vi "EndTest_WithTime_DurationIsSet.vi"() -> (0 "error out":errorcluster)   [LabVIEW 2017, in "ResultTreeListenerTest.lvlib"]
uses:
  ResultTreeListenerTest.lvlib
  ResultTreeListener/ResultTreeListener.lvclass
  ResultTree/ResultTree.lvclass
  Support/FakeTestCase/FakeTestCase.lvclass
  C:/Users/de200256/Code/neuperger/lvunit/Test/Test.lvclass
  275d98eb-69a7-4435-8809-2af3ffd1cf1d.vi
panel:
  in  "Tree":string(tree)
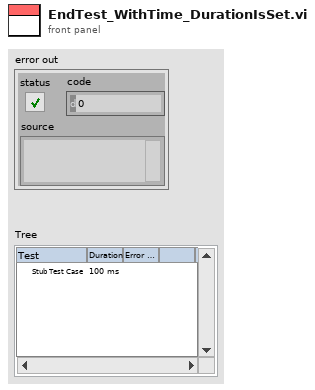
[diagram p1: front panel]
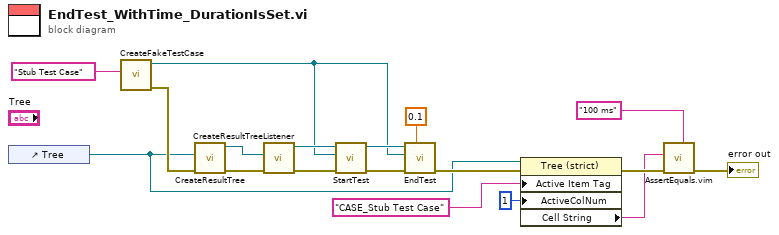
[diagram p0: block diagram]
diagram:
  n1 = control-ref of="Tree"() -> (w5:refnum<vi>)
  n2 = call "CreateFakeTestCase.vi"("Name"="Stub Test Case") -> ("error out"=w10:errorcluster, "FakeTestCase out"=w8:refnum<class "FakeTestCase.lvclass">)  [unwired: 9 in]
  n3 = call "CreateResultTree.vi"("error in (no error)"=w10, "Tree Refnum"=w5) -> ("error out"=w18:errorcluster, "ResultTree out"=w17:refnum<class "ResultTree.lvclass">)  [unwired: 8 in]
  n4 = call "CreateResultTreeListener.vi"("error in (no error)"=w18, "ResultTree"=w17) -> ("error out"=w16:errorcluster, "ResultTreeListener out"=w14:refnum<class "ResultTreeListener.lvclass">)  [unwired: 8 in]
  n5 = call-dynamic "StartTest.vi"("error in (no error)"=w16, "Test"=w8, "ResultTreeListener in"=w14) -> ("error out"=w12:errorcluster, "ResultTreeListener out"=w11:refnum<class "ResultTreeListener.lvclass">)  [unwired: 7 in]
  n6 = call-dynamic "EndTest.vi"("Time"=0.1, "error in (no error)"=w12, "Test"=w8, "ResultTreeListener in"=w11) -> ("error out"=w9:errorcluster)  [unwired: 6 in, 1 out]
  n7 = property class="Tree (strict)"(reference=w5, error in=w9, "Active Item Tag"="CASE_Stub Test Case" ("Active Item:Tag"), "ActiveColNum"=1 ("Active Cell:Active Column Number")) -> (error out=w6:errorcluster, "Cell String"=w1:string)  [unwired: 1 out]
  n8 = call "AssertEquals.vim"("Expected"="100 ms" ("Active Cell:String"), "error in (no error)"=w6, "Actual"=w1) -> ("error out"=→"error out":errorcluster)  [unwired: 8 in]
